vi "Init.vi"(0 "IV in":refnum<class "IV.lvclass">, 5 "Path":path, 7 "IV_meas.lvclass":refnum<class "IV_meas.lvclass">, 9 "IV_data.lvclass":refnum<class "IV_data.lvclass">, 11 "error in (no error)":errorcluster) -> (4 "IV out":refnum<class "IV.lvclass">, 15 "error out":errorcluster)   [LabVIEW 2014, in "IV.lvclass"]
uses:
  IV.lvclass
  meas/IV_meas.lvclass
  data/IV_data.lvclass
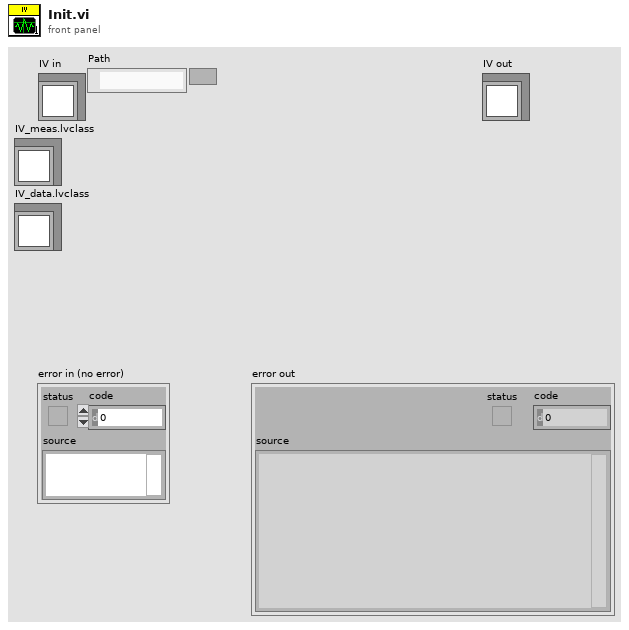
[diagram p1: front panel]
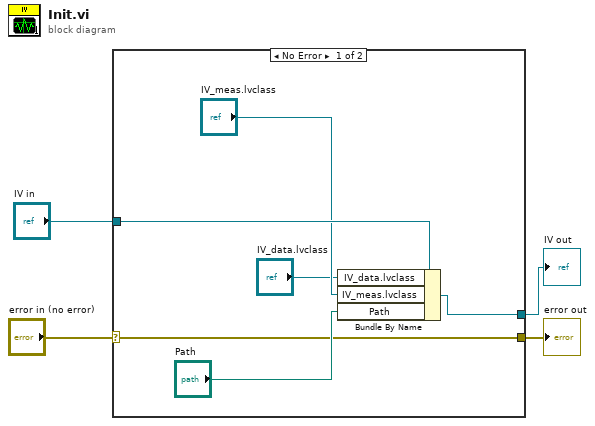
[diagram p0: block diagram]
diagram:
  n1 = case shown="No Error" "error in (no error)" {
    selector: "error in (no error)" -> [w6 w12]
    tunnel: [w6 w12] -> w3
    tunnel: "IV in" -> [w10 w11]
    tunnel: [w7 w11] -> w1
    frame No Error {
      n2 = Bundle By Name(cluster=w10, "IV_data.lvclass"="IV_data.lvclass", "IV_meas.lvclass"="IV_meas.lvclass", "Path"="Path") -> (w7:refnum<class "IV.lvclass">)
    }
    frame Error {
    }
  }
  "error out" <- w3
  "IV out" <- w1
